vi "_prebuild_federate_interface.vi"() -> ()   [LabVIEW 2016]
uses:
  support/controls/prebuild_federate_interface_actions.ctl
  support/controls/raw_object_interaction_descriptor.ctl
panel:
  out "loaded_content":string
  out "lib_path":path
  out "status":string
  out "cancelled":bool
  out "error out":errorcluster
  in  "error in (no error)":errorcluster
  # "Instructions:\n\n(1) open the project this VI is a part of\n(2) re-open this VI (if opened prior to opening the owning project)\n(3) run the VI\n(4) follow the prompts\n\nWhat to Expect:\n\nThis utility VI is intended take as input a complete FOM.xml\nfile and output a \"federate library\" of auto-generated LabVIEW\ncode to a target directory of choosing.  It is suggested to opt for\nthe default location (within this LabVIEW project) as it can be\neasily referenced from other independent projects.\n\nWhat to expect.  This utility prompts for the location of a FOM.xml\nfile.  That file is then digested and parsed for all possible objects\nand interactions in the federate model this xml file is intended\nto represent.  It then outputs to a \"federate_library\" directory a\nseries of strict type clusters, one for each of the interactions and/or\nobjects parsed from the FOM.xml.\n\nAdditionally, two major \"queues\" are generated.  One queue names\n\"incoming_queue.vi\" shall be used within a custom written LabVIEW\nprogram for receiving incoming object or interaction based notifications\nfrom the HLA network being subscribed to.\n\nThe \"outgoing_queue\" in turn outputs any updates to interactions and/or\nobjects associated with the federate model.  Fortunately, these interactions\nand/or objects (as mentioned above) live as LabVIEW clusters for ease\nof interfacing."
  # "Builder Status"
  # "Loaded content"
  # "Federate Library Build Location"
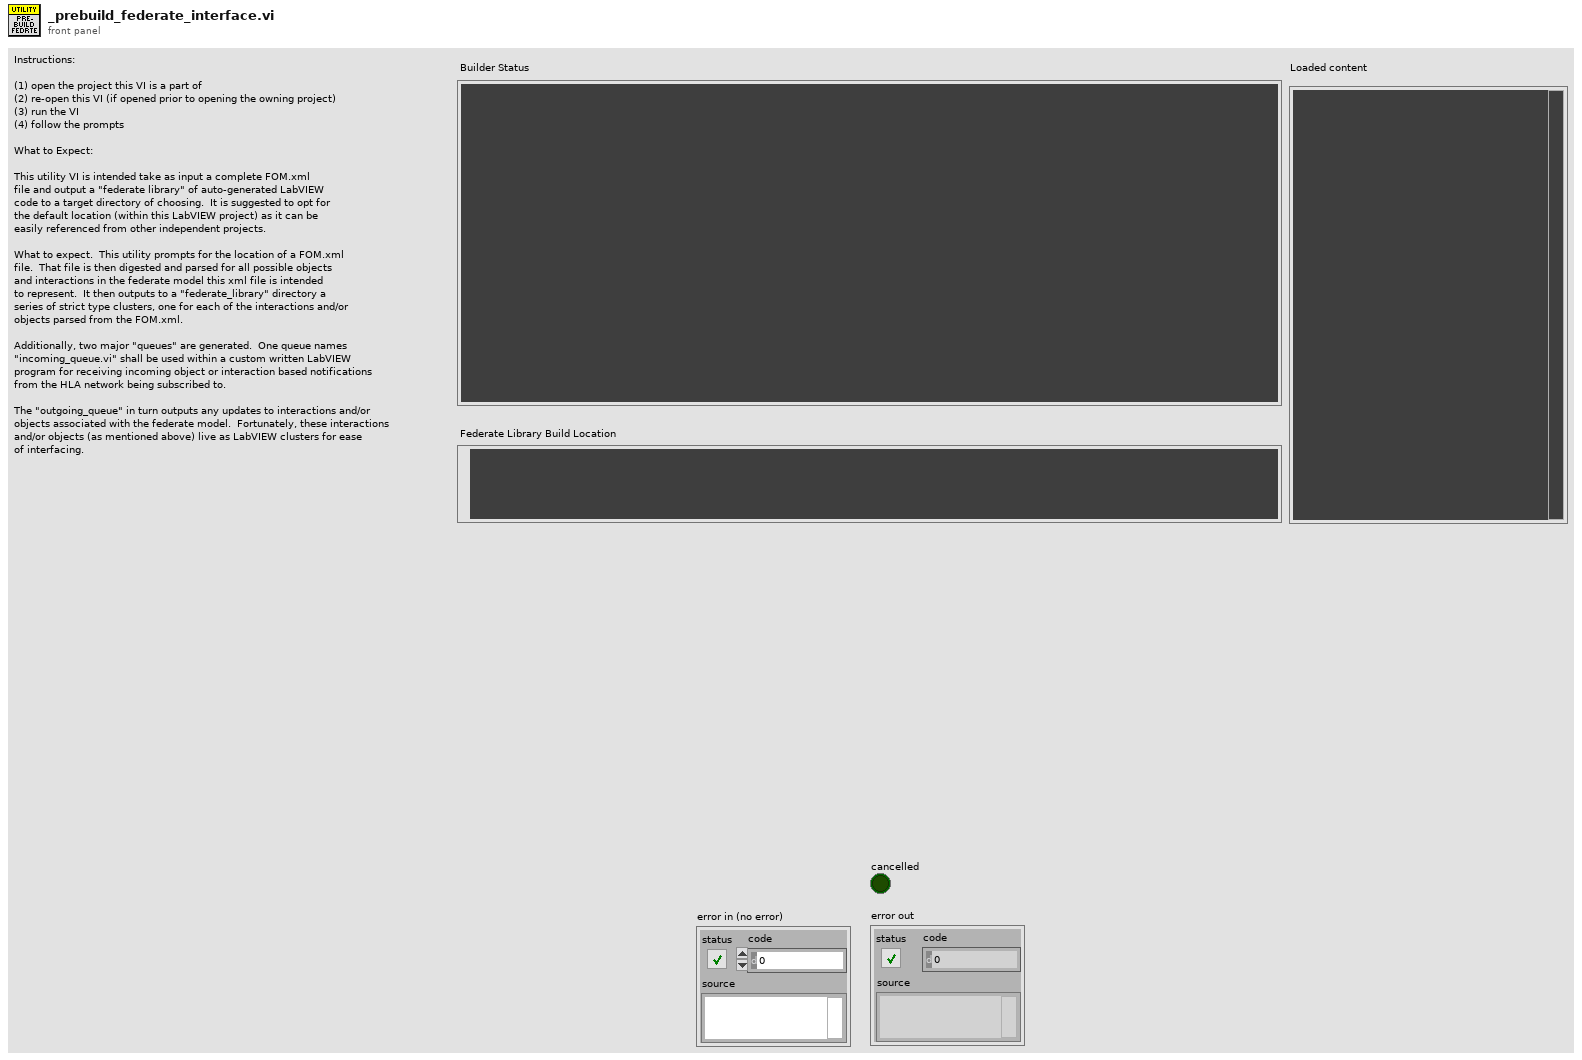
[diagram p1: front panel]
types:
  T1 = typedef "prebuild_federate_interface_actions.ctl" = enum16{"build_clusters", "build_poly_queues", "choose_interface_directory", "init", "load_fom"}
  T2 = enum32{"invalid app kind", "Development System", "Run Time System", "Student Edition", "Embedded LabVIEW", "Evaluation", "Custom"}
  T3 = typedef "raw_object_interaction_descriptor.ctl" = cluster{"classpath (id)":string, "shortname":string, "param_names":string[], "param_dtypes":string[]}
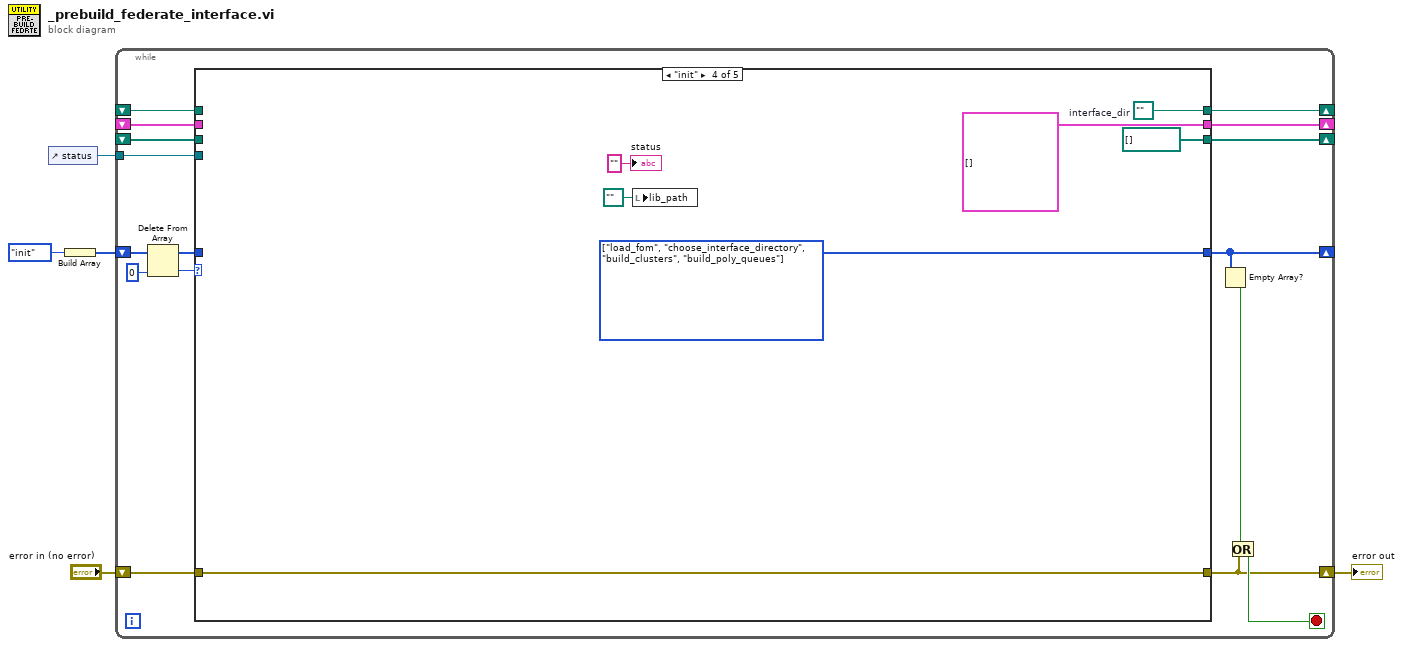
[diagram p0: block diagram]
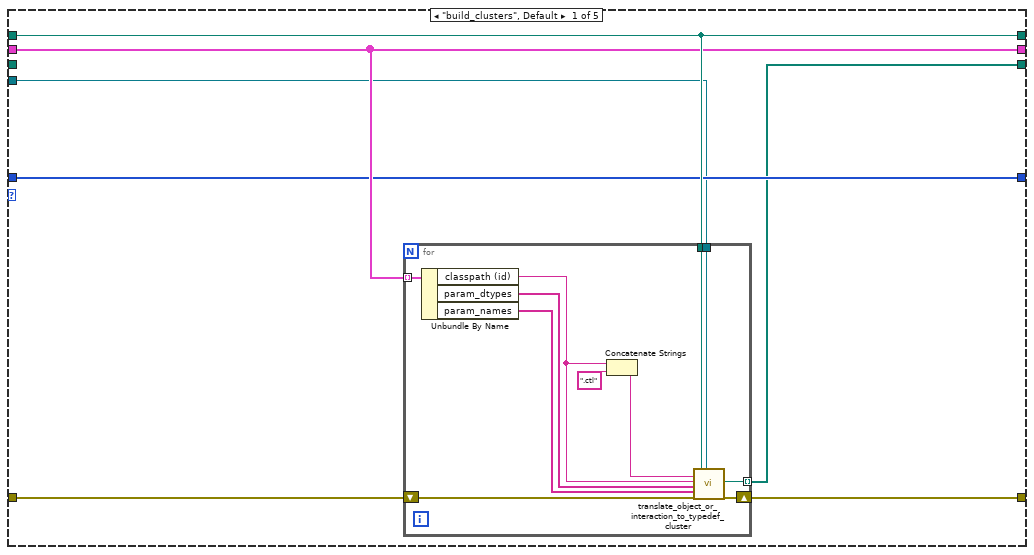
[diagram p2: hidden frame]
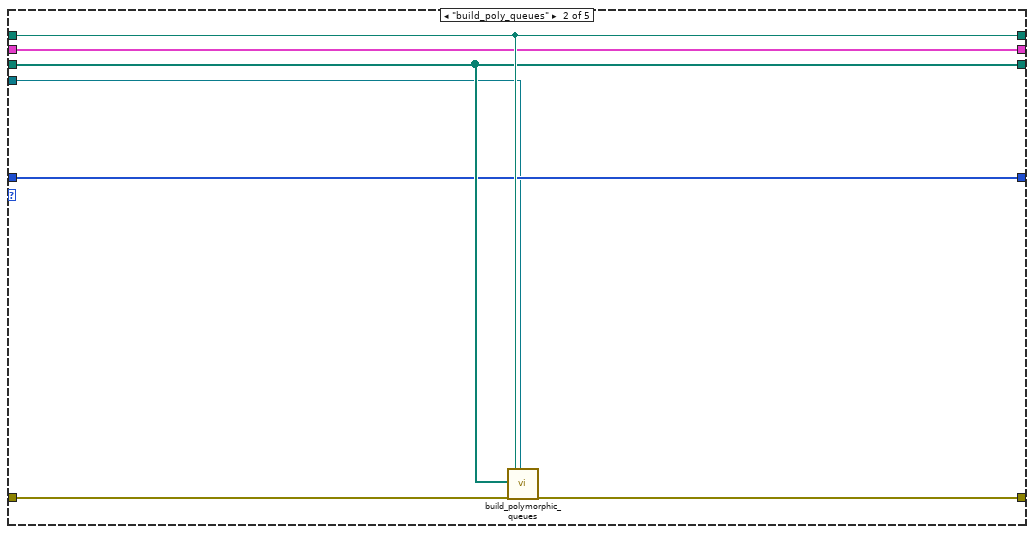
[diagram p3: hidden frame]
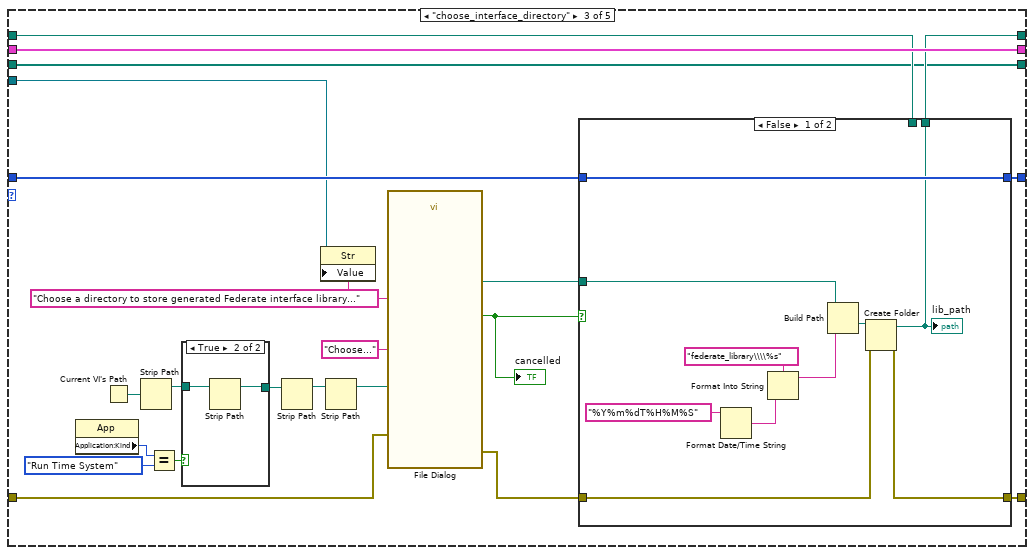
[diagram p4: hidden frame]
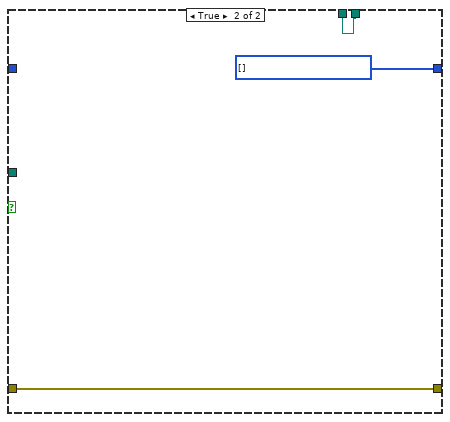
[diagram p6: hidden frame]
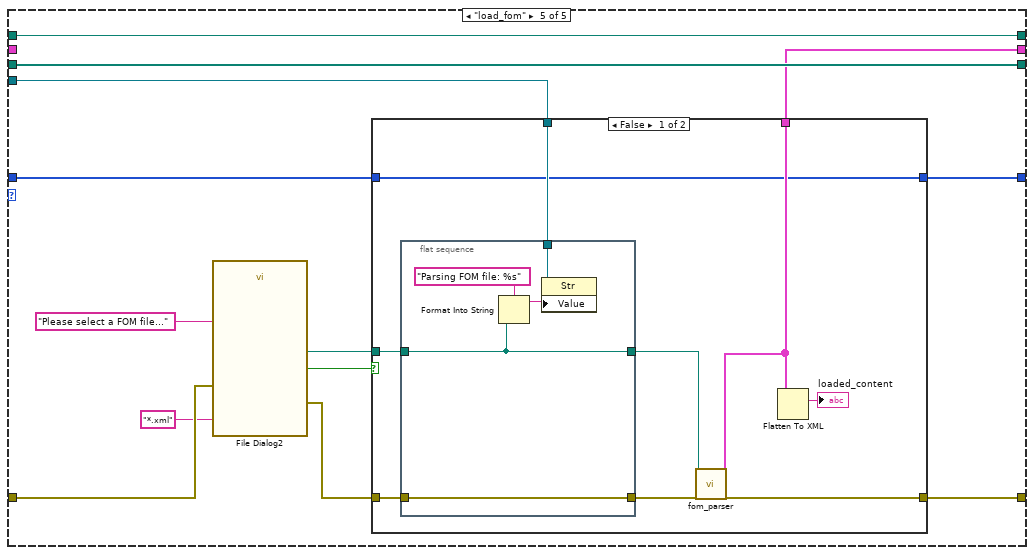
[diagram p7: hidden frame]
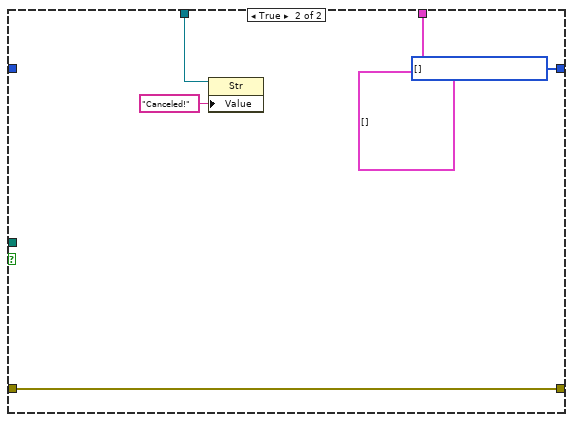
[diagram p8: hidden frame]
diagram:
  n1 = control-ref of="status"() -> (w1:refnum<vi>)
  n2 = Build Array(prebuild_federate_interface_actions."init" ("actions")) -> (w4:T1[])
  n3 = while {
    shift-right: [w17] -> _
    shift-left: w4 -> [w21]
    shift-right: [w13] -> w2
    shift-left: "error in (no error)" -> [w16]
    shift-right: [w12] -> _
    shift-left: _ -> [w11]
    shift-right: [w10] -> _
    shift-left: _ -> [w9]
    shift-right: [w8] -> _
    shift-left: _ -> [w7]
    tunnel: w1 -> [w6]
    stop <- w14 stop-if-true
    n4 = Delete From Array(array=w21, index=0) -> (deleted portion=w19:T1, array with subset deleted=w18:T1[])  [unwired: 1 in]
    n5 = case shown="\"init\"" w19 {
      tunnel: w18 -> [w24 w41 w65 _ w95]
      tunnel: [w24 w41 w64 w91 w94] -> w17
      tunnel: [w27 w45 w62 w88 w102] -> w13
      tunnel: w16 -> [w28 w46 w68 w88 w98]
      tunnel: [w26 w44 w59 w90 w104] -> w12
      tunnel: w11 -> [w26 w44 w58 _ w104]
      tunnel: [w25 w43 w63 T3[] [] w100] -> w10
      tunnel: w9 -> [w25 w43 w63 _ _]
      tunnel: [w23 w42 w57 path[] [] w103] -> w8
      tunnel: w7 -> [_ w42 w57 _ w103]
      tunnel: w6 -> [w22 w40 w56 _ w101]
      frame "build_clusters", Default {
        n6 = for {
          shift-right: [w38] -> w27
          shift-left: w28 -> [w39]
          tunnel: w25 -> [w36] mode=indexing
          tunnel: w26 -> [w37]
          tunnel: [w30] -> w23 mode=indexing
          tunnel: w22 -> [w29]
          n7 = Unbundle By Name(w36) -> ("classpath (id)"=w33:string, "param_dtypes"=w35:string[], "param_names"=w34:string[])
          n8 = Concatenate Strings(w33, ".ctl" ("string")) -> (w31:string)
          n9 = call "translate_object_or_interaction_to_typedef_cluster.vi"("typedef_control_name (in)"=w31, "item_classpath (in)"=w33, "datatypes (in)"=w35, "attribute_names (in)"=w34, "error in (no error)"=w39, "base_federate_dir (in)"=w37, "status_ref (in)"=w29) -> ("saved_typedef (out)"=w30:path, "error out"=w38:errorcluster)  [unwired: 11 in]
        }
      }
      frame "build_poly_queues" {
        n10 = call "build_polymorphic_queues.vi"("object/interaction_cluster_paths (in)"=w42, "error in (no error)"=w46, "base_federate_dir (in)"=w44, "status_ref (in)"=w40) -> ("error out"=w45:errorcluster)  [unwired: 15 in]
      }
      frame "choose_interface_directory" {
        w55 = "Choose a directory to store generated Federate interface library..." ("prompt")
        n11 = property on="Property Node" class="App"() -> ("Application:Kind"=w53:T2)  [unwired: 2 in, 2 out]
        n12 = Current VI's Path() -> (path=w54:path)
        n13 = Strip Path(path=w54) -> (stripped path=w50:path)  [unwired: 1 out]
        n14 = Equal?(x=w53, y=T2."Run Time System") -> (x = y?=w51:bool)
        n15 = case shown="True" w51 {
          tunnel: w50 -> [w69 w71]
          tunnel: [w69 w70] -> w49
          frame False {
          }
          frame True {
            n16 = Strip Path(path=w71) -> (stripped path=w70:path)  [unwired: 1 out]
          }
        }
        n17 = Strip Path(path=w49) -> (stripped path=w48:path)  [unwired: 1 out]
        n18 = property class="Str"(reference=w56, "Value"=w55) -> ()  [unwired: 1 in, 2 out]
        n19 = Strip Path(path=w48) -> (stripped path=w47:path)  [unwired: 1 out]
        n20 = call "File Dialog"("start path"=w47, "prompt"=w55, "button label"="Choose...", "error in"=w68) -> ("selected path"=w60:path, "cancelled"=w66:bool, "error out"=w61:errorcluster)  [unwired: 8 in, 1 out]
        "cancelled" <- w66
        n21 = case shown="False" w66 {
          tunnel: w65 -> [w81 _]
          tunnel: [w81 w84] -> w64
          tunnel: w61 -> [w74 w83]
          tunnel: [w73 w83] -> w62
          tunnel: w60 -> [w80 _]
          tunnel: [w72 w82] -> w59
          tunnel: w58 -> [_ w82]
          frame False {
            n22 = Format Date/Time String(time format string (%c)="%Y%m%dT%H%M%S") -> (date/time string=w76:string)  [unwired: 2 in]
            n23 = Format Into String(format string="federate_library\\\\%s" ("name or relative path"), w76) -> (resulting string=w75:string)  [unwired: 2 in, 1 out]
            n24 = Build Path(base path=w80, name or relative path=w75) -> (appended path=w79:path)
            n25 = Create Folder(path (use dialog)=w79, error in=w74) -> (created path=w72:path, error out=w73:errorcluster)  [unwired: 1 in, 1 out]
            "lib_path" <- w72
          }
          frame True {
            w84 = T1[] [] items=["build_clusters", "build_poly_queues", "choose_interface_directory", "init", "load_fom"]
          }
        }
      }
      frame "init" {
        w90 = path ""  # interface_dir
        w91 = T1[] [enum."load_fom", enum."choose_interface_directory", enum."build_clusters", enum."build_poly_queues"] items=["build_clusters", "build_poly_queues", "choose_interface_directory", "init", "load_fom"]
        n26 = local write "lib_path"(path "" ("lib_path")) -> ()
        "status" <- "" ("status")
      }
      frame "load_fom" {
        n27 = call "File Dialog2"("prompt"="Please select a FOM file...", "error in"=w98, "pattern (all files)"="*.xml") -> ("selected path"=w96:path, "cancelled"=w93:bool, "error out"=w97:errorcluster)  [unwired: 9 in, 1 out]
        n28 = case shown="False" w93 {
          tunnel: [w113 w121] -> w102
          tunnel: w101 -> [w111 w120]
          tunnel: [w108 T3[] [] ("items (out)")] -> w100
          tunnel: w97 -> [w107 w121]
          tunnel: w96 -> [w106 _]
          tunnel: w95 -> [w105 _]
          tunnel: [w105 w123] -> w94
          frame False {
            n29 = flat-sequence {
              tunnel: w111 -> [w118]
              tunnel: w106 -> [w114]
              tunnel: [w115] -> w110
              tunnel: w107 -> [w115]
              tunnel: [w114] -> w109
              frame #0 {
                n30 = Format Into String(format string="Parsing FOM file: %s", w114) -> (resulting string=w116:string)  [unwired: 2 in, 1 out]
                n31 = property class="Str"(reference=w118, "Value"=w116) -> ()  [unwired: 1 in, 2 out]
              }
            }
            n32 = call "fom_parser.vi"("fom_path (in)"=w109, "error in (no error)"=w110) -> ("interaction_descriptors (out)"=w108:T3[], "error out"=w113:errorcluster)  [unwired: 16 in]
            n33 = Flatten To XML(anything=w108) -> (xml string=→"loaded_content":string)
          }
          frame True {
            w123 = T1[] [] items=["build_clusters", "build_poly_queues", "choose_interface_directory", "init", "load_fom"]
            n34 = property class="Str"(reference=w120, "Value"="Canceled!") -> ()  [unwired: 1 in, 2 out]
          }
        }
      }
    }
    n35 = Empty Array?(array=w17) -> (empty?=w15:bool)
    n36 = Or(x=w15, y=w13) -> (x .or. y?=w14:bool)
  }
  "error out" <- w2
